vi "Set TargetVelocity.vi"(8 "error in (no error)":errorcluster, 11 "Value":sgl=9.0) -> (0 "error out":errorcluster)   [LabVIEW 2020, in "输出轴伺服.lvlib"]
uses:
  Servo_global.vi
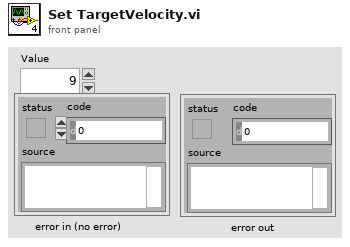
[diagram p1: front panel]
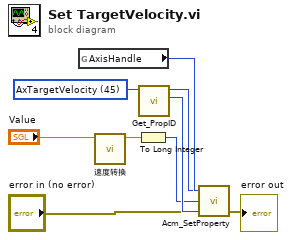
[diagram p0: block diagram]
diagram:
  w7 = u16 45 items=["AxTargetPosition"=44, "AxTargetVelocity"=45, "AxTargetTorque"=46, "AxControlWord"=47, "AxStatusWord"=48, "AxOperationMode"=49, "AxMaxTorque"=333] ("Prop")
  n1 = global read "Servo_global.vi" "AxisHandle"() -> (w9:u32)
  n2 = call "速度转换.vi"("In"="Value") -> ("Out"=w2:sgl)  [unwired: 10 in]
  n3 = To Long Integer(number=w2) -> (32bit integer=w1:i32)
  n4 = call "Get_PropID.vi"("Prop"=w7) -> ("BufferLength"=w6:u32, "PropID"=w8:u32)  [unwired: 9 in]
  n5 = call <userlib>:"Acm_SetProperty.vi"("Handle"=w9, "ProperyID"=w8, "Buffer"=w1, "Error Input(No Error)"="error in (no error)", "BufferLength"=w6) -> ("Error Output"=→"error out":errorcluster)  [unwired: 2 out]
